vi "(8) part 2 que.vi"(10 "Numeric in":dbl, 11 "Numeric 3":dbl) -> (3 "Numeric out":dbl)   [LabVIEW 2025]
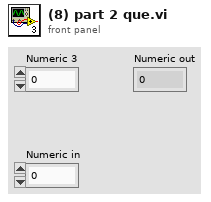
[diagram p1: front panel]
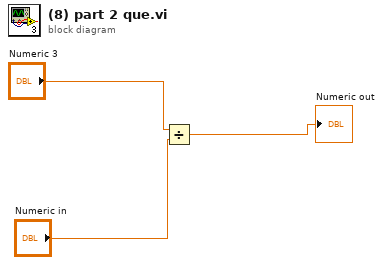
[diagram p0: block diagram]
diagram:
  n1 = Divide(x="Numeric 3", y="Numeric in") -> (x/y=→"Numeric out":dbl)
